vi "from string 3.3.vi"(8 "error in":errorcluster, 10 "data in":string, 11 "Shared Memory configuration in":refnum<class "Shared Memory configuration.lvclass">) -> (0 "error out":errorcluster, 2 "remaining data":string, 3 "Shared Memory configuration out":refnum<class "Shared Memory configuration.lvclass">)   [LabVIEW 2013, in "Shared Memory configuration.lvclass"]
uses:
  Shared Memory configuration.lvclass
  Shared Memory configuration.lvclass/Shared Memory configuration.ctl
  <vilib>/NI/Configuration Framework/serializable configuration/NISE_CEF_serializable configuration.lvclass
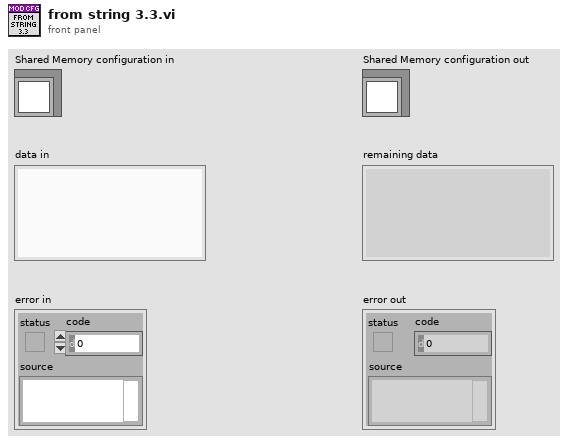
[diagram p1: front panel]
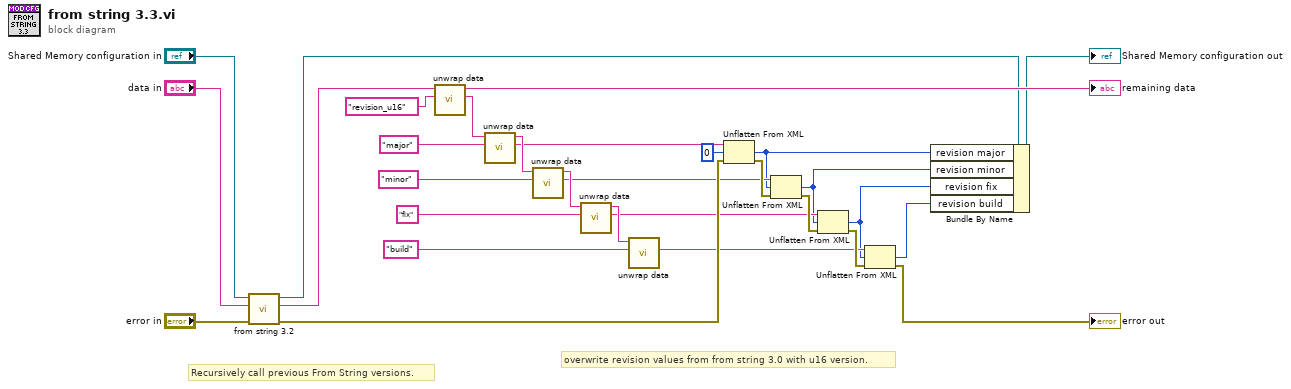
[diagram p0: block diagram]
diagram:
  # "overwrite revision values from from string 3.0 with u16 version."
  # "Recursively call previous From String versions."
  n1 = call "from string 3.2.vi"("error in"="error in", "data in"="data in", "Shared Memory configuration in"="Shared Memory configuration in") -> ("error out"=w30:errorcluster, "remaining data"=w23:string, "Shared Memory configuration out"=w25:refnum<class "Shared Memory configuration.lvclass">)  [unwired: 6 in]
  n2 = call <vilib>:"unwrap data.vi"("identifier"="revision_u16", "data to unwrap"=w23) -> ("unwrapped data"=w15:string, "remaining string"=→"remaining data":string)  [unwired: 8 in]
  n3 = call <vilib>:"unwrap data.vi"("identifier"="major", "data to unwrap"=w15) -> ("unwrapped data"=w10:string, "remaining string"=w18:string)  [unwired: 8 in]
  n4 = call <vilib>:"unwrap data.vi"("identifier"="minor", "data to unwrap"=w18) -> ("unwrapped data"=w9:string, "remaining string"=w17:string)  [unwired: 8 in]
  n5 = call <vilib>:"unwrap data.vi"("identifier"="fix", "data to unwrap"=w17) -> ("unwrapped data"=w8:string, "remaining string"=w16:string)  [unwired: 8 in]
  n6 = call <vilib>:"unwrap data.vi"("identifier"="build", "data to unwrap"=w16) -> ("unwrapped data"=w7:string)  [unwired: 8 in, 1 out]
  n7 = Unflatten From XML(xml string=w10, type=u16 0, error in (no error)=w30) -> (value=w6:u16, error out=w14:errorcluster)
  n8 = Unflatten From XML(xml string=w9, type=w6, error in (no error)=w14) -> (value=w5:u16, error out=w13:errorcluster)
  n9 = Unflatten From XML(xml string=w8, type=w5, error in (no error)=w13) -> (value=w4:u16, error out=w12:errorcluster)
  n10 = Unflatten From XML(xml string=w7, type=w4, error in (no error)=w12) -> (value=w3:u16, error out=→"error out":errorcluster)
  n11 = Bundle By Name(cluster=w25, "revision major"=w6, "revision minor"=w5, "revision fix"=w4, "revision build"=w3) -> (→"Shared Memory configuration out":refnum<class "Shared Memory configuration.lvclass">)
